vi "Get Palette Menu Information Demo.vi"() -> ()   [LabVIEW 2022 SP3]
uses:
  System.Drawing
panel:
  in  "Back":bool
  in  "Array":T1(array[cluster])
  in  "Palette Menu Path":path
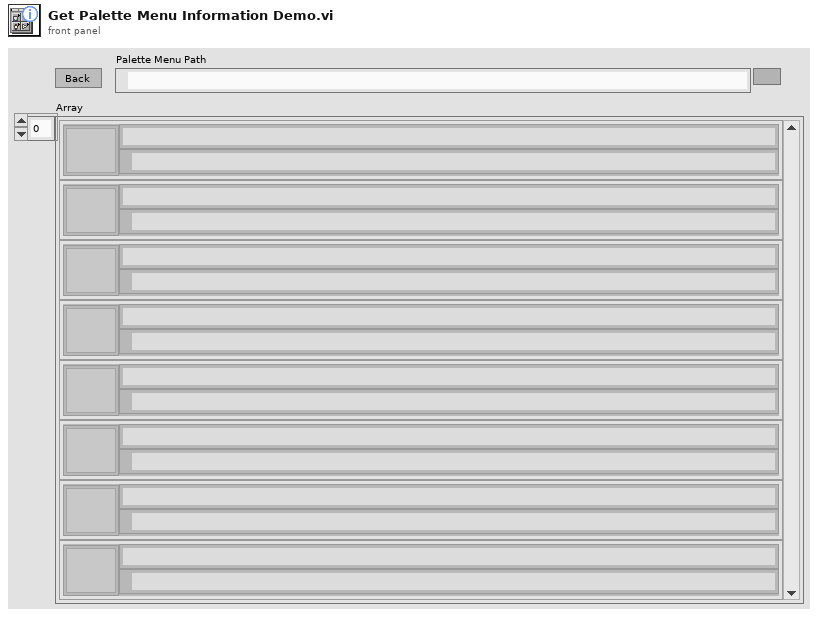
[diagram p1: front panel]
types:
  T1 = cluster{"Name":string, "Path":path, "Icon":picture, "Btn":bool}[]
  T2 = cluster{"Item name":string, "file path":path, "new picture":picture, "Btn":bool}
  T3 = cluster{"Name":string, "Path":path, "Icon":picture, "Btn":bool}
  T4 = cluster{"Palette Item Type":enum32{"Submenu", "VI", "Express VI", "Built In", "Empty"}, "short name":string, "Item name":string, "file path":path, "image":u8[]}[]
  T5 = typedef "imagedata.ctl" = cluster{"image type":i32, "image depth":i32, "image":u8[], "mask":u8[], "colors":u32[], "Rectangle":cluster{"left":i16, "top":i16, "right":i16, "bottom":i16}}
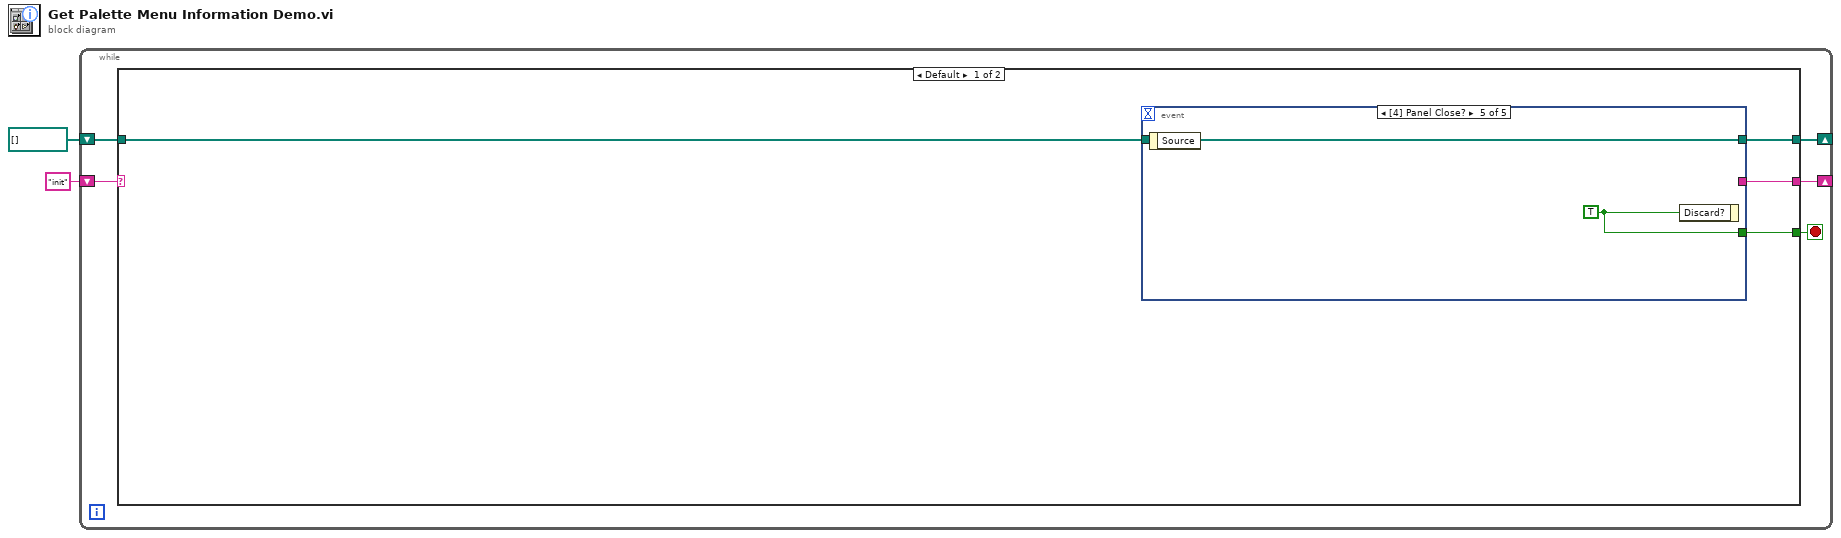
[diagram p0: block diagram]
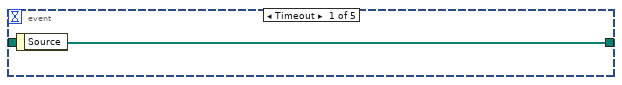
[diagram p2: hidden frame]
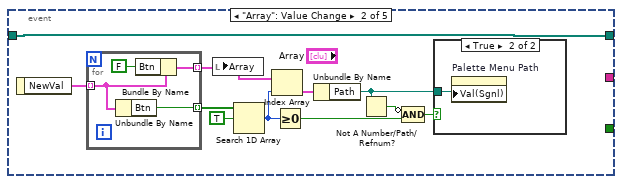
[diagram p3: hidden frame]
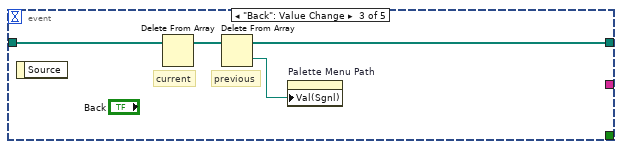
[diagram p5: hidden frame]
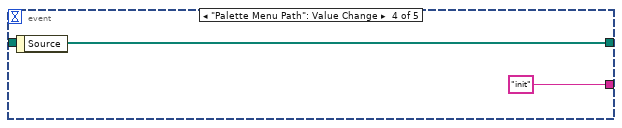
[diagram p6: hidden frame]
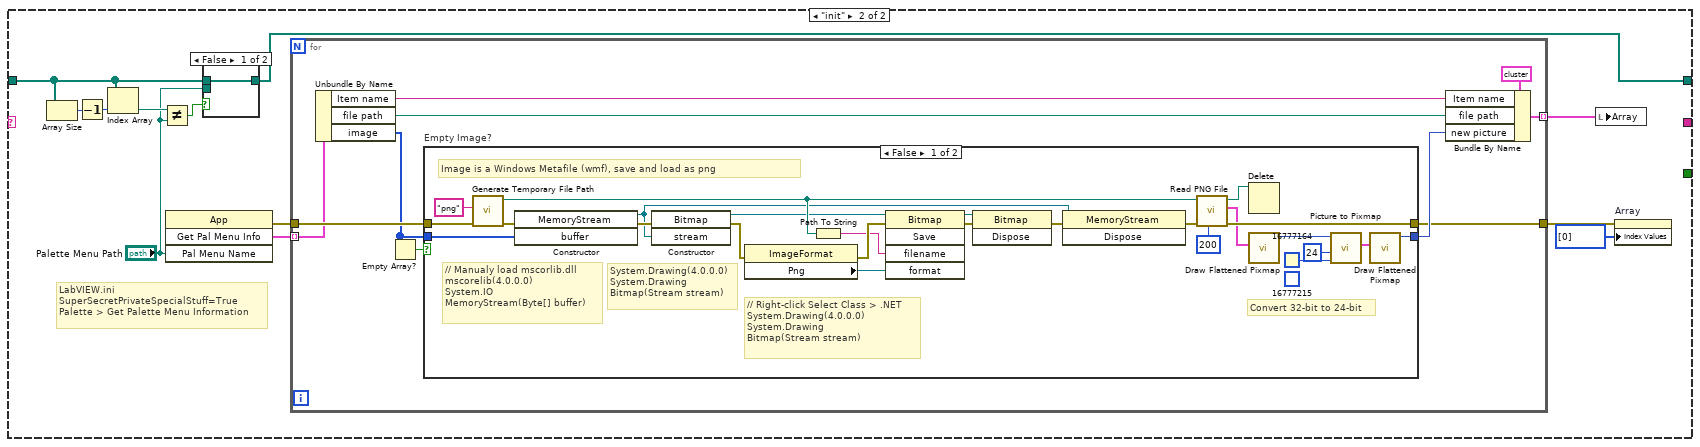
[diagram p7: hidden frame]
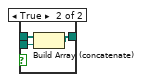
[diagram p8: hidden frame]
diagram:
  n1 = while {
    shift-right: [w6] -> _
    shift-left: "init" -> [w7]
    shift-right: [w3] -> _
    shift-left: path[] [] -> [w4]
    stop <- w5 stop-if-true
    n2 = case shown="Default" w7 {
      tunnel: [w11 _] -> w6
      tunnel: [w10 _] -> w5
      tunnel: w4 -> [w9 w44]
      tunnel: [w8 w45] -> w3
      frame Default {
        n3 = event shown="[4] Panel Close?" {
          selector: _ -> [_ _ _ _ _]
          dyn-events: _ -> [_ _ _ _ _]
          timeout: _ -> [_ _ _ _ _]
          tunnel: [_ _ _ "init" _] -> w11
          tunnel: [_ _ _ _ w36] -> w10
          tunnel: w9 -> [w12 w16 w31 w33 w35]
          tunnel: [w12 w16 w30 w33 w35] -> w8
          event Timeout {
            n4 = event-data() -> ()  [unwired: 1 in, 1 out]
          }
          event "Array": Value Change {
            n5 = event-data() -> ("NewVal"=w23:T1)  [unwired: 1 in]
            n6 = for {
              tunnel: w23 -> [w27] mode=indexing
              tunnel: [w28] -> w22 mode=indexing
              tunnel: [w25] -> w20 mode=indexing
              n7 = Unbundle By Name(w27) -> ("Btn"=w28:bool)
              n8 = Bundle By Name(cluster=w27, "Btn"=FALSE) -> (w25:T3)
            }
            n9 = local write "Array"(w20) -> ()
            n10 = Search 1D Array(1D array=w22, element=TRUE) -> (index of element=w18:i32)  [unwired: 1 in]
            n11 = Index Array(array=w20, index=w18) -> (element=w19:T3)
            n12 = Greater Or Equal To 0?(x=w18) -> (x >= 0?=w17:bool)
            n13 = Unbundle By Name(w19) -> ("Path"=w15:path)
            n14 = Not A Number/Path/Refnum?(number/path/refnum=w15) -> (NaN/Path/Refnum?=w13:bool)
            n15 = Compound Arithmetic op=AND(invert w13, w17) -> (w14:bool)
            n16 = case shown="True" w14 {
              tunnel: w15 -> [_ w24]
              frame False {
              }
              frame True {
                n17 = property on="Palette Menu Path" class="Path"("Val(Sgnl)"=w24) -> ()  [unwired: 2 in, 2 out]
              }
            }
          }
          event "Back": Value Change {
            # "previous"
            # "current"
            n18 = event-data() -> ()  [unwired: 1 in, 1 out]
            n19 = Delete From Array(array=w31) -> (array with subset deleted=w32:path[])  [unwired: 2 in, 1 out]
            n20 = Delete From Array(array=w32) -> (deleted portion=w29:path, array with subset deleted=w30:path[])  [unwired: 2 in]
            n21 = property on="Palette Menu Path" class="Path"("Val(Sgnl)"=w29) -> ()  [unwired: 2 in, 2 out]
          }
          event "Palette Menu Path": Value Change {
            n22 = event-data() -> ()  [unwired: 1 in, 1 out]
          }
          event Panel Close? {
            w36 = TRUE ("Discard?")
            n23 = event-data() -> ()  [unwired: 1 in, 1 out]
            n24 = event-data("Discard?"=w36) -> ()  [unwired: 1 in, 1 out]
          }
        }
      }
      frame "init" {
        # "LabVIEW.ini\nSuperSecretPrivateSpecialStuff=True\nPalette > Get Palette Menu Information"
        n25 = Array Size(array=w44) -> (size(s)=w43:i32)
        n26 = Decrement(x=w43) -> (x-1=w42:i32)
        n27 = Index Array(array=w44, index=w42) -> (element=w41:path)
        n28 = Not Equal?(x=w41, y="Palette Menu Path") -> (x != y?=w39:bool)
        n29 = invoke class="App" method="Get Pal Menu Info"("Pal Menu Name"="Palette Menu Path") -> (error out=w48:errorcluster, "Get Palette Menu Info"=w47:T4)  [unwired: 3 in, 2 out]
        n30 = case shown="False" w39 {
          tunnel: [w49 w52] -> w45
          tunnel: w44 -> [w49 w51]
          tunnel: "Palette Menu Path" -> [_ w50]
          frame False {
          }
          frame True {
            n31 = Build Array (concatenate)(w51, w50) -> (w52:path[])
          }
        }
        n32 = for {
          tunnel: w48 -> [w61]
          tunnel: w47 -> [w60] mode=indexing
          tunnel: [w54] -> w46 mode=indexing
          tunnel: [w53] -> w37
          n33 = Unbundle By Name(w60) -> ("Item name"=w58:string, "file path"=w57:path, "image"=w59:u8[])
          n34 = Empty Array?(array=w59) -> (empty?=w62:bool)
          n35 = case "Empty Image?" shown="False" w62 {
            tunnel: w59 -> [w87 _]
            tunnel: [w80 w88] -> w53
            tunnel: w61 -> [w79 w88]
            tunnel: [w63 _] -> w56
            frame False {
              (unwired) u32 16777215 ("Background Color")
              # "Convert 32-bit to 24-bit"
              # "Image is a Windows Metafile (wmf), save and load as png"
              # "// Right-click Select Class > .NET\nSystem.Drawing(4.0.0.0)\nSystem.Drawing\nBitmap(Stream stream)"
              # "System.Drawing(4.0.0.0)\nSystem.Drawing\nBitmap(Stream stream)"
              # "// Manualy load mscorlib.dll\nmscorelib(4.0.0.0)\nSystem.IO\nMemoryStream(Byte[] buffer)"
              n36 = call <vilib>:"Generate Temporary File Path.vi"("error in (no error)"=w79, "Temporary File Extension (tmp)"="png") -> ("error out"=w78:errorcluster, "Unique Temporary File Path"=w76:path)  [unwired: 8 in]
              n37 = constructor class="MemoryStream"(error in=w78, "buffer"=w87) -> (reference out=w70:refnum<k24>, error out=w86:errorcluster)  [unwired: 2 in, 2 out]
              n38 = constructor class="Bitmap"(error in=w86, "stream"=w70) -> (reference out=w65:refnum<k24>, error out=w83:errorcluster)  [unwired: 2 in, 2 out]
              n39 = property class="ImageFormat"(error in=w83) -> (error out=w82:errorcluster, "Png"=w74:refnum<k24>)  [unwired: 1 in, 1 out]
              n40 = Path To String(path=w76) -> (string=w69:string)
              n41 = invoke class="Bitmap" method="Save"(reference=w65, error in=w82, "filename"=w69, "format"=w74) -> (reference out=w85:refnum<k24>, error out=w84:errorcluster)  [unwired: 1 in, 3 out]
              n42 = invoke class="Bitmap" method="Dispose"(reference=w85, error in=w84) -> (error out=w68:errorcluster)  [unwired: 1 in, 2 out]
              n43 = invoke class="MemoryStream" method="Dispose"(reference=w70, error in=w68) -> (error out=w81:errorcluster)  [unwired: 1 in, 2 out]
              n44 = call <vilib>:"Read PNG File.vi"("Transparency Thresh"=u8 200, "error in (no error)"=w81, "path to PNG file"=w76) -> ("error out"=w80:errorcluster, "image data"=w66:T5, "path"=w75:path)  [unwired: 6 in]
              n45 = Delete(path (use dialog)=w75) -> ()  [unwired: 4 in, 3 out]
              n46 = call <vilib>:"Draw Flattened Pixmap.vi"("image data"=w66) -> ("new picture"=w73:picture)  [unwired: 8 in]
              n47 = call <vilib>:"Picture to Pixmap.vi"("Background Color"=u32 16777164, "depth"=24, "picture"=w73) -> ("image data"=w64:T5)  [unwired: 7 in, 1 out]
              n48 = call <vilib>:"Draw Flattened Pixmap.vi"("image data"=w64) -> ("new picture"=w63:picture)  [unwired: 8 in]
            }
            frame True {
            }
          }
          n49 = Bundle By Name(cluster=T2 {"Item name"="", "file path"=path "", "new picture"=bytes[0], "Btn"=FALSE}, "Item name"=w58, "file path"=w57, "new picture"=w56) -> (w54:T2)
        }
        n50 = local write "Array"(w46) -> ()
        n51 = property on="Array" class="Arr (strict)"(error in=w37, "Index Values"=u32[] [0]) -> ()  [unwired: 1 in, 2 out]
      }
    }
  }
